vi "Система_ТП-ГРЩ-ЩАХП.vi"() -> ()   [LabVIEW 2016]
panel:
  out "АХП\nдистанц.\nупр-е":bool
  in  "Дистанц.\nупр.\nАХП":bool
  out "АВАРИЯ":bool
  out "УКРМ\nВВОД 2":bool
  out "УКРМ\nВВОД 1":bool
  in  "Авария\nВВОД 2":bool
  in  "Авария\nВВОД  2":bool
  out "АВР\nВВОД  2":bool
  out "АВР\nВВОД 1":bool
  out "I 0.4 кВ ВВОД 2, А":i64(knob) scale=0.0..630.0
  out "U 0.4 кВ ВВОД 2, В":i64(knob) scale=340.0..420.0
  out "I 0.4 кВ ВВОД 1, А":i64(knob) scale=0.0..630.0
  out "U 0.4 кВ ВВОД 1, В":i64(knob) scale=340.0..420.0
  in  "Вкл. РЗиА\nВВОД2":bool
  in  "Вкл. РЗиА\nВВОД1":bool
  out "I 10 кВ ВВОД 2, А":i64(knob) scale=0.0..630.0
  out "U 10 кВ ВВОД 2, В":i64(knob) scale=9000.0..11000.0
  out "I 10 кВ ВВОД 1, А":i64(knob) scale=0.0..630.0
  out "U 10 кВ ВВОД 1, В":i64(knob) scale=9000.0..11000.0
  out "АХП\nреле\nвремени":bool
  in  "Вкл.\nтаймера":bool
  out "Текущее время":string
  out "Текущая дата":string
  in  "Целевле время":string
  in  "Целевая дата":string
  # "Кнопки с индикацией РЗиА выполняют фунцию по остановке системы, для\nимитации аварии по стороне высокого напряжения, с целью последующего\nперезапуска системы в ручном режме. Генерация токов и напряжений \nосуществляется рандом, синусоиду и осцилограмму включать в программу \nпосчитал нецелесообразным. Цикличность  - время задержки в мс, отражается \nна работу всего цикла. Значение 1000, тк при использовании глобальных\nпеременных у меня не получилось синхронизировать работу циклов."
  # "Копки с индикацией Авария выполняют функцию по включению АВР между двумя вводами, в случае отключения по двум вводам включается красный сигнал АВАРИЯ. В случае генерации напряжения и тока хотя бы по одному из вводов и, если включено дистанционное управвление - включается индикатор АХП, который имитирует включение групп архитектурной подсветки. Индикаторы УКРМ включены, когда соответвующий ввод находится в рабочем состоянии."
  # "<= Проводит сверку введеной целевой даты с текущим. Если true то включает \nиндикатор АХП. Время включения - 1000 мс, из-за рассинхронизации\nкак раз и не смог запустить на регулируемое длительное значение."
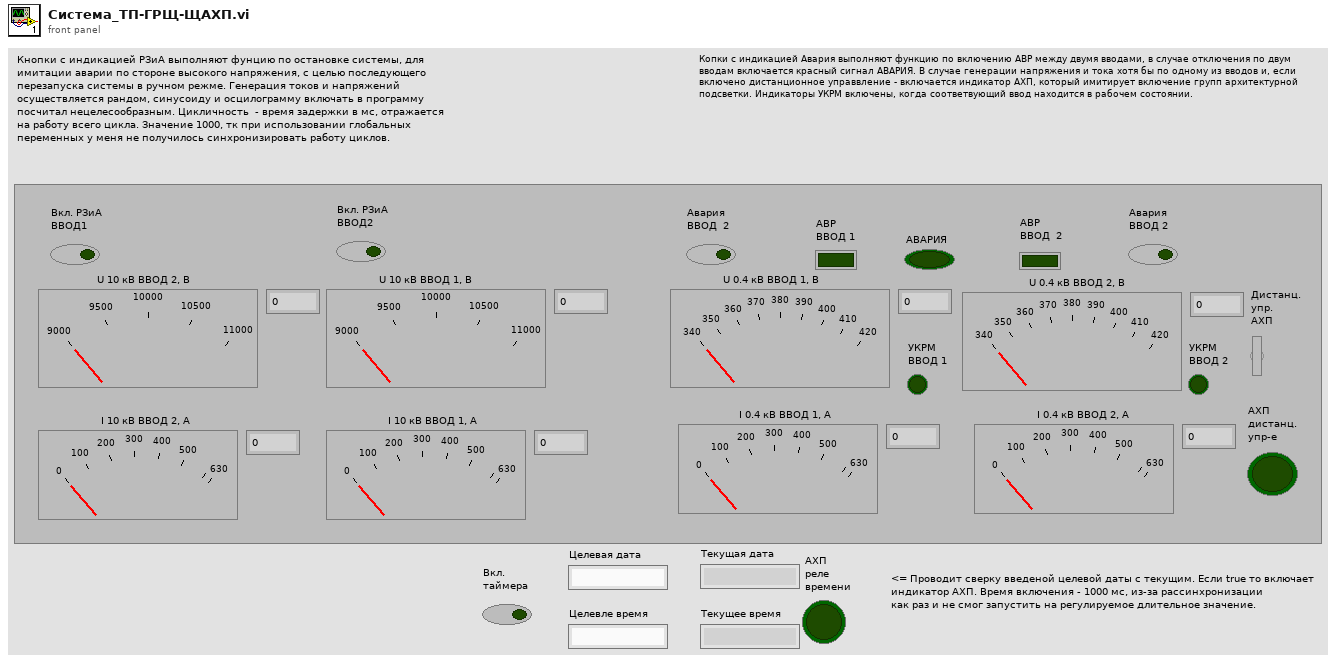
[diagram p1: front panel]
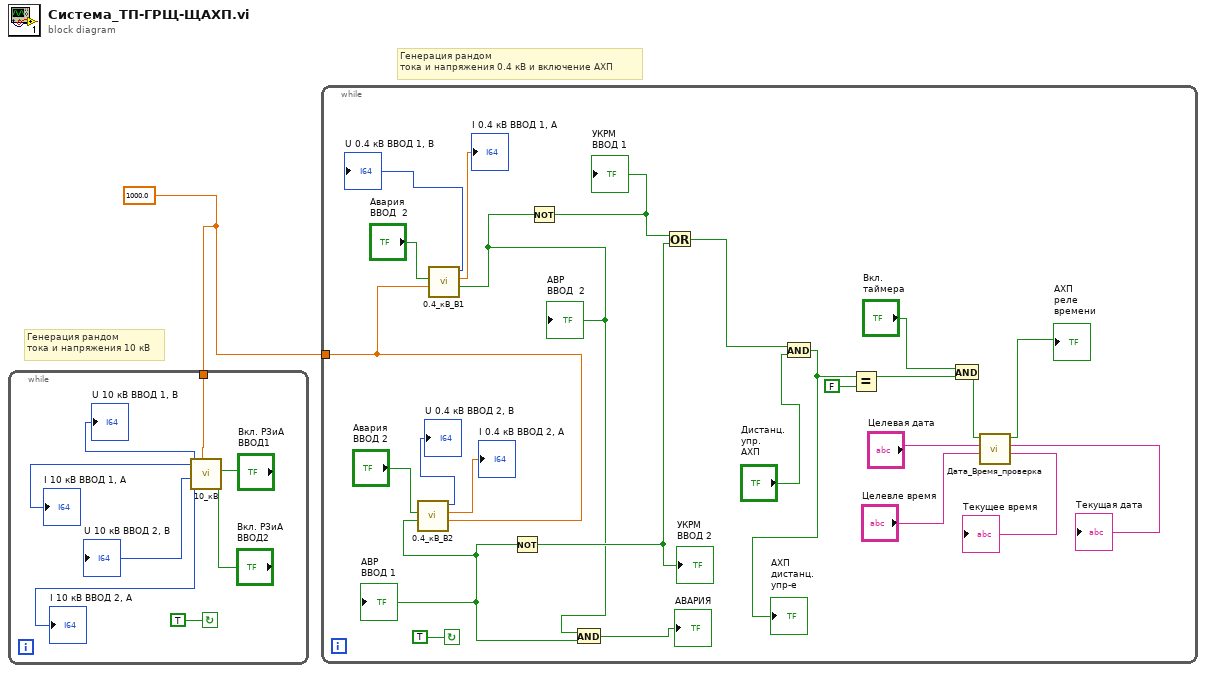
[diagram p0: block diagram]
diagram:
  w1 = 1000.0 ("Цикличность  2")
  # "Генерация рандом\nтока и напряжения 0.4 кВ и включение АХП"
  # "Генерация рандом\nтока и напряжения 10 кВ"
  n1 = while {
    tunnel: w1 -> [w4]
    stop <- TRUE continue-if-true
    n2 = call "10_кВ.vi"("Вкл. РЗиА 2"="Вкл. РЗиА\nВВОД2", "Вкл. РЗиА 1"="Вкл. РЗиА\nВВОД1", "Time\ndelay"=w4) -> ("I 10 кВ ВВОД 2"=→"I 10 кВ ВВОД 2, А":i64, "U 10 кВ ВВОД 2"=→"U 10 кВ ВВОД 2, В":i64, "I 10 кВ ВВОД 1"=→"I 10 кВ ВВОД 1, А":i64, "U 10 кВ ВВОД 1"=→"U 10 кВ ВВОД 1, В":i64)  [unwired: 3 in, 2 out]
  }
  n3 = while {
    tunnel: w1 -> [w25]
    stop <- TRUE continue-if-true
    n4 = call "0.4_кВ_В2.vi"("Time delay"=w25, "Авария ВВОД 1"="Авария\nВВОД 2") -> ("АВР\nВВОД 2"=w27:bool, "Амперметр 0,4 кВ ВВОД 2"=→"I 0.4 кВ ВВОД 2, А":dbl, "Вольтметр 0,4 кВ ВВОД 2"=→"U 0.4 кВ ВВОД 2, В":i64)  [unwired: 7 in]
    "АВР\nВВОД 1" <- w27
    n5 = call "0.4_кВ_В1.vi"("Time delay"=w25, "Авария ВВОД 1"="Авария\nВВОД  2") -> ("АВР\nВВОД1 2"=w32:bool, "Амперметр 0,4 кВ ВВОД1 2"=→"I 0.4 кВ ВВОД 1, А":dbl, "Вольтметр 0,4 кВ ВВОД 2"=→"U 0.4 кВ ВВОД 1, В":i64)  [unwired: 6 in]
    "АВР\nВВОД  2" <- w32
    n6 = Not(x=w27) -> (.not. x?=w33:bool)
    "УКРМ\nВВОД 2" <- w33
    n7 = Not(x=w32) -> (.not. x?=w23:bool)
    "УКРМ\nВВОД 1" <- w23
    n8 = And(x=w32, y=w27) -> (x .and. y?=→"АВАРИЯ":bool)
    n9 = Or(x=w23, y=w33) -> (x .or. y?=w20:bool)
    n10 = And(x=w20, y="Дистанц.\nупр.\nАХП") -> (x .and. y?=w14:bool)
    "АХП\nдистанц.\nупр-е" <- w14
    n11 = Equal?(x=w14, y=FALSE) -> (x = y?=w11:bool)
    n12 = And(x="Вкл.\nтаймера", y=w11) -> (x .and. y?=w10:bool)
    n13 = call "Дата_Время_проверка.vi"("Целевое время"="Целевле время", "Целевая дата"="Целевая дата", "Boolean 2"=w10) -> ("Текущее время"=→"Текущее время":string, "Текущая дата"=→"Текущая дата":string, "Boolean"=→"АХП\nреле\nвремени":bool)  [unwired: 6 in]
  }
